vi "ReceiveSendDataReferenceResponse.vi"(8 "error in (no error)":errorcluster, 11 "body":variant) -> (0 "error out":errorcluster, 1 "error code":i32, 3 "event reference":T1, 4 "error info":string)   [LabVIEW 2017, in "ServerComm.lvlib"]
doc: "Parses the Send Data Reference Response message."
uses:
  <vilib>/addons/InsightCM/Devices/Shared/Common/ServerComm/ServerComm.lvlib
  <vilib>/addons/InsightCM/Devices/Shared/Common/DataEvent/controls/EventReference.ctl
  <vilib>/addons/InsightCM/Devices/Shared/Common/DataEvent/controls/Event.ctl
  <vilib>/addons/InsightCM/MessageBus/Base/controls/DataEvent.ctl
  <vilib>/addons/InsightCM/MessageBus/Base/controls/KeyValuePair.ctl
  <vilib>/addons/InsightCM/Devices/Shared/Common/DataEvent/controls/DataSet.ctl
  <vilib>/addons/InsightCM/MessageBus/Base/controls/DataSetMetadata.ctl
  <vilib>/addons/InsightCM/MessageBus/Base/controls/TrendPoint.ctl
  <vilib>/addons/InsightCM/MessageBus/Base/controls/TrendAlarmUpdate.ctl
  <vilib>/addons/InsightCM/MessageBus/Base/controls/TrendAlarmTransition.ctl
  <vilib>/addons/InsightCM/Devices/Shared/Common/ServerComm/controls/SendDataEvent.ctl
  <vilib>/addons/InsightCM/Devices/Shared/Common/DataEvent/DataEvent.lvlib
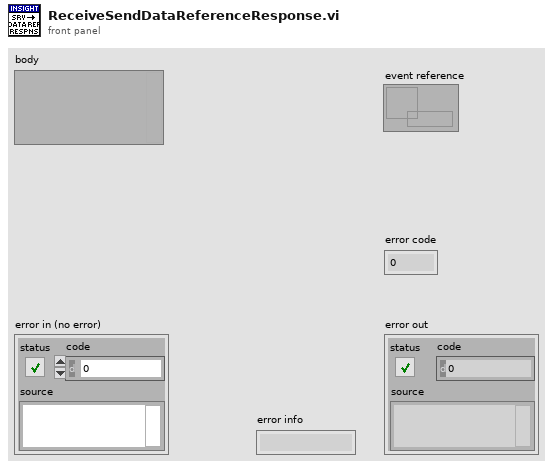
[diagram p1: front panel]
types:
  T1 = typedef "DataEvent.lvlib/EventReference.ctl" = refnum<data-value>
  T2 = typedef "ServerComm.lvlib/SendDataEvent.ctl" = cluster{"event reference":T1, "StreamId":string, "Block":i32, "Properties":T3[]}
  T3 = typedef "KeyValuePair.ctl" = cluster{"Key":string, "Value":string}
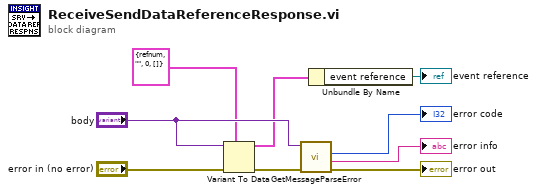
[diagram p0: block diagram]
diagram:
  n1 = Variant To Data(error in="error in (no error)", type=T2 {"event reference"=refnum, "StreamId"="", "Block"=0, "Properties"=[]} ("Body"), Variant="body") -> (data=w3:T2, error out=w8:errorcluster)
  n2 = call <vilib>:"GetMessageParseError.vi"("error in (no error)"=w8, "body"="body") -> ("error out"=→"error out":errorcluster, "error info"=→"error info":string, "error code"=→"error code":i32)  [unwired: 7 in]
  n3 = Unbundle By Name(w3) -> ("event reference"=→"event reference":T1)
